vi "1-Tap 8-bit Camera with Bayer (FPGA).vi"() -> ()   [LabVIEW 2012]
doc: "This is the FPGA VI for the 1-Tap 8-Bit Camera with Bayer example. This example demonstrates how to acquire images from a 1-tap, 8-bit, base configuration, Camera Link camera, with a color sensor and transfer the decoded images to the host via a DMA FIFO.\n\nThis example also demonstrates the use of third-party IP imported into the LabVIEW project as a CLIP. In this case, the imported CLIP comes from an FPGA netlist and performs the Bayer color decoding to convert the incoming 8-bit Bayer images into 24-bit RGB images in real time.\n\nAdditionally, the example demonstrates the serial server, which allows third-party camera configuration utilities to communicate with the camera using the Camera Link serial interface while this VI is running."
uses:
  Common/CL Signal Mapping.ctl
  Common/CL Configuration.ctl
  <vilib>/Platform/TimedLoop/XDataNode/timing_clust.ctl
  <vilib>/Platform/TimedLoop/XDataNode/nitl_modes.ctl
  <vilib>/Platform/TimedLoop/XDataNode/wakeup.ctl
  <vilib>/rvi/eio/common/nirviEmuTemplateMethod_errors.vi
  <vilib>/rvi/Emulation/niFpgaSctlEmulationRegisterWithScheduler.vi
  <vilib>/rvi/Emulation/niFpgaSctlEmulationScheduler.vi
  Common/CL Data to Pixels/1 Tap 8-Bit.vi
  <vilib>/rvi/interface/RandomDataEmulation/nirviRandomDataFPGAFIFO.vi
  <vilib>/rvi/interface/RandomDataEmulation/niFpgaRandomDataHandleErrors.vi
  <vilib>/rvi/Emulation/niFpgaSctlEmulationGlobalWrite.vi
  <vilib>/Platform/TimedLoop/XDataNode/XDataNode.xnode
  <vilib>/eio/EIONode/EIONode.xnode
  <vilib>/rvi/DataTransferAndStorage/Container/XNode/niFpgaContainer.xnode
  <vilib>/rvi/interface/RandomDataEmulation/nirviRandomDataFpgaReadWriteTemplate.vi
  <vilib>/Platform/TimedLoop/XDataNode/XDNodeRunTimeDep.lvlib
panel:
  in  "CL Config.Configuration":T1
  in  "CL Config.Signal Mapping":T2
  in  "CL Config.Line Scan":bool
  in  "CL Config.DVAL Active High":bool=TRUE
  in  "CL Config.LVAL Active High":bool=TRUE
  in  "CL Config.FVAL Active High":bool=TRUE
  in  "CL Config.Spare Active High":bool=TRUE
  in  "Bayer Decoder.Image Width":u16
  in  "Bayer Decoder.First Column Is Red":bool
  in  "Bayer Decoder.First Row Is Blue":bool
  in  "Acq Control.Line Scan Height":u32
  in  "Acq Control.Frames To Acq":u32
  in  "Acq Control.Acquire":bool
  in  "Acq Control.Cancel Acq":bool
  in  "Acq Control.Ignore DVAL":bool
  in  "Acq Control.Initialize":bool
  out "Acq Status.Acq In Progress":bool
  out "Acq Status.Clocks Per Line":u32
  out "Acq Status.Frames Acq'd":u32
  out "Acq Status.Lines Per Frame":u32
  out "Acq Status.DMA Write Timeout":bool
  out "Acq Status.Initialized":bool
  in  "UART.Baud Rate":u8
  in  "UART.Transmit":bool
  in  "UART.Tx Data":u8[](array[numeric])=[0, 0, 0, 0, 0, 0, 0, 0, 0, 0] format="%02x"
  in  "UART.Set Baud Rate":bool
  in  "UART.Byte Mode":bool=TRUE
  out "UART.Rx Ready":bool
  out "UART.Break Indicator":bool
  out "UART.Framing Error":bool
  out "UART.Overrun Error":bool
  out "UART.Tx Ready":bool
  out "UART.Rx Data":u8 format="%02x"
  in  "UART.Receive":bool
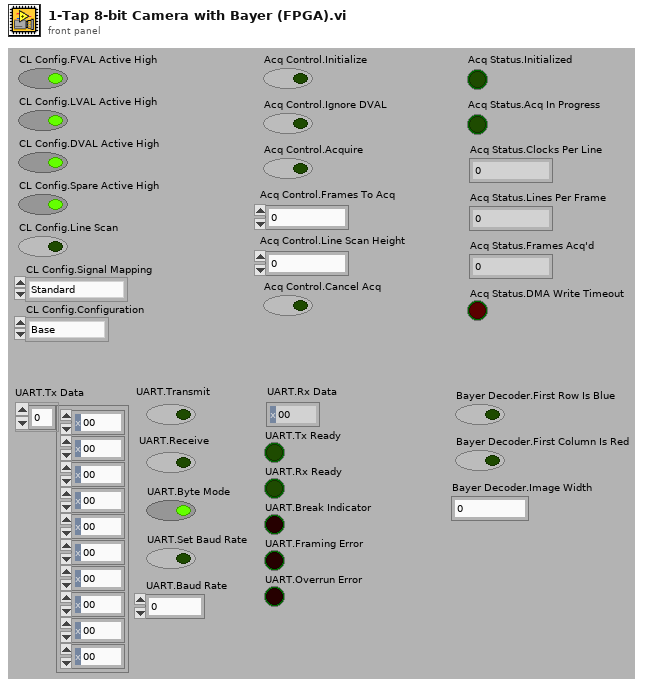
[diagram p1: front panel]
types:
  T1 = typedef "CL Configuration.ctl" = enum8{"Base", "Medium", "Full"}
  T2 = typedef "CL Signal Mapping.ctl" = enum8{"Standard", "Basler 10-tap", "Vosskühler 10-tap"}
  T3 = typedef "XDNodeRunTimeDep.lvlib/timing_clust.ctl" = cluster{"Expected End [f-1]":u64, "Actual End [f-1]":u64, "Finished Late? [f-1]":bool, "Expected End [i-1]":u64, "Actual End [i-1]":u64, "Finished Late? [i-1]":bool, "Expected Start [i]":u64, "Actual Start [i]":u64, "Expected Start [f]":u64, "Actual Start [f]":u64, "Source Name":string, "Structure Name":string, "Period":i64, "Deadline":i64, "Offset":i64, "Start":i64, "Priority":i32, "Timeout":i32, "Mode":T4, "Wakeup Reason":T5, "Error":errorcluster, "Source Type":string, "Secondary Source Type":string, "Global End Time":u64, "Global Start Time":u64, "Frame Duration":u64, "Iteration Duration":u64, "Assigned CPU":i32, "I/O Scan Engine Mode":u32}
  T4 = typedef "XDNodeRunTimeDep.lvlib/nitl_modes.ctl" = enum32{"No Change", "Process missed periods, maintain original phase", "Discard missed periods, maintain original phase", "Process missed periods, ignore original phase", "Discard missed periods, ignore original phase"}
  T5 = typedef "XDNodeRunTimeDep.lvlib/wakeup.ctl" = enum32{"Normal", "Aborted", "Asynchronous wakeup", "Timing source error", "Timed loop error", "Timeout"}
  T6 = cluster{"Enables Valid":bool, "Frame Valid":bool, "Line Valid":bool, "Data Valid":bool}
  T7 = cluster{"Tx Data":u8[], "Transmit":bool, "Receive":bool, "Byte Mode":bool, "Set Baud Rate":bool, "Baud Rate":u8}
  T8 = cluster{"Rx Data":u8, "Turn Off Transmit":bool, "Turn Off Receive":bool, "Turn Off Set Baud Rate":bool, "Tx Ready":bool, "Rx Ready":bool, "Break Indicator":bool, "Framing Error":bool, "Overrun Error":bool}
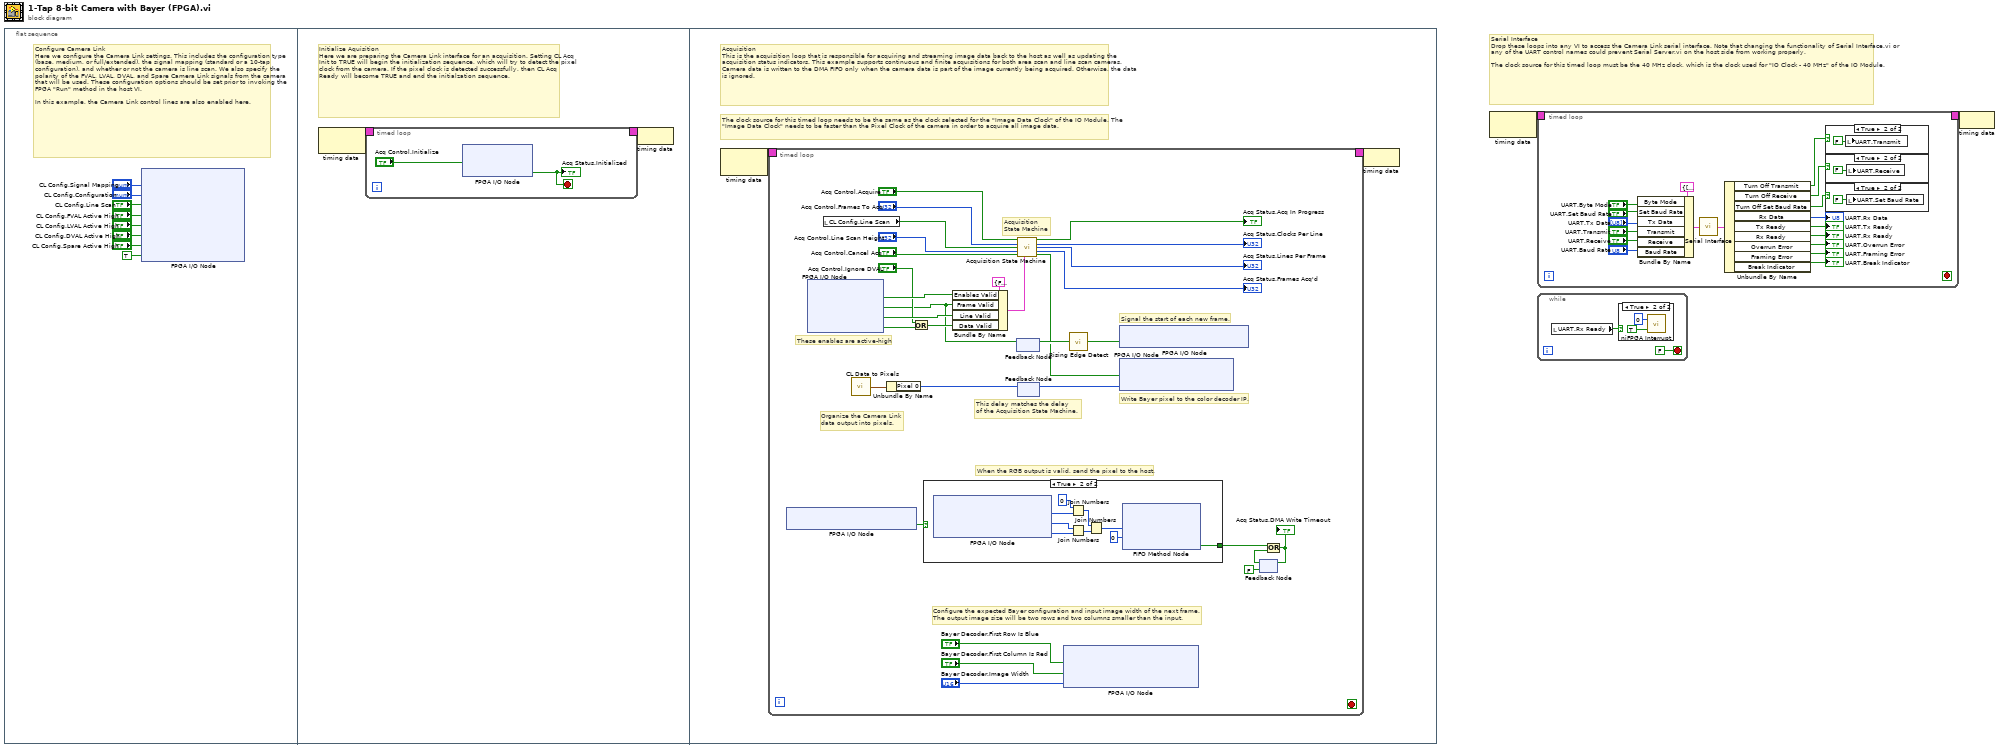
[diagram p0: block diagram]
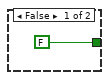
[diagram p6: hidden frame]
diagram:
  # "Serial Interface\nDrop these loops into any VI to access the Camera Link serial interface. Note that changing the functionality of Serial Interface.vi or any of the UART control names could prevent Serial Server.vi on the host side from working properly.\n\nThe clock source for this timed loop must be the 40 MHz clock, which is the clock used for \"IO Clock - 40 MHz\" of the IO Module."
  n1 = flat-sequence {
    frame #0 {
      # "Configure Camera Link\nHere we configure the Camera Link settings. This includes the configuration type (base, medium, or full/extended), the signal mapping (standard or a 10-tap configuration), and whether or not the camera is line scan. We also specify the polarity of the FVAL, LVAL, DVAL, and Spare Camera Link signals from the camera that will be used. These configuration options should be set prior to invoking the FPGA \"Run\" method in the host VI.\n\nIn this example, the Camera Link control lines are also enabled here."
      n2 = xnode "FPGA I/O Node"("CL Set Signal Mapping"="CL Config.Signal Mapping", "CL Set Configuration"="CL Config.Configuration", "CL Set Line Scan"="CL Config.Line Scan", "CL Set FVAL Active High"="CL Config.FVAL Active High", "CL Set LVAL Active High"="CL Config.LVAL Active High", "CL Set DVAL Active High"="CL Config.DVAL Active High", "CL Set Spare Active High"="CL Config.Spare Active High", "CL Control Enable"=TRUE ("IO Module\\CL Control Enable")) -> ()  [unwired: 8 in, 8 out]
    }
    frame #1 {
      # "Initialize Aquisition\nHere we are preparing the Camera Link interface for an acquisition. Setting CL Acq Init to TRUE will begin the initialization sequence, which will try to detect the pixel clock from the camera. If the pixel clock is detected successfully, then CL Acq Ready will become TRUE and end the initialzation sequence."
      n3 = node-c288() -> (w12:T3)  [unwired: 1 out]
      n4 = timed-loop {
        timing: w12 -> [_]
        timing-out: [_] -> w11
        stop <- w13 stop-if-true
        n5 = xnode "FPGA I/O Node"("CL Acq Init"="Acq Control.Initialize") -> ("CL Acq Ready"=w13:bool)  [unwired: 2 in, 2 out]
        "Acq Status.Initialized" <- w13
      }
      n6 = node-c288(w11) -> ()
    }
    frame #2 {
      # "The clock source for this timed loop needs to be the same as the clock selected for the \"Image Data Clock\" of the IO Module. The \"Image Data Clock\" needs to be faster than the Pixel Clock of the camera in order to acquire all image data."
      # "Acquisition\nThis is the acquisition loop that is responsible for acquiring and streaming image data back to the host as well as updating the acquisition status indicators. This example supports continuous and finite acquisitions for both area scan and line scan cameras. Camera data is written to the DMA FIFO only when the camera data is part of the image currently being acquired. Otherwise, the data is ignored."
      n7 = node-c288() -> (w20:T3)  [unwired: 1 in]
      n8 = timed-loop {
        timing: w20 -> [_]
        timing-out: [_] -> w19
        stop <- _ stop-if-true
        # "Configure the expected Bayer configuration and input image width of the next frame.\nThe output image size will be two rows and two columns smaller than the input."
        # "When the RGB output is valid, send the pixel to the host."
        # "Write Bayer pixel to the color decoder IP."
        # "Signal the start of each new frame."
        # "Organize the Camera Link\ndata output into pixels."
        # "These enables are active-high"
        # "This delay matches the delay\nof the Acquisition State Machine."
        # "Acquisition\nState Machine"
        n9 = xnode "FPGA I/O Node"() -> ("Bayer Decoder\\RGB Output Valid"=w30:bool)  [unwired: 1 in, 1 out]
        n10 = xnode "FPGA I/O Node"() -> ("CL Output Valid"=w39:bool, "CL Frame Valid"=w27:bool, "CL Line Valid"=w38:bool, "CL Data Valid"=w35:bool)  [unwired: 4 in, 4 out]
        n11 = local read "CL Config.Line Scan"() -> (w32:bool)
        n12 = call-poly "CL Data to Pixels.vi"() -> ("Pixels"=w51:cluster{"Pixel 0":u8})  [unwired: 1 in]
        n13 = Unbundle By Name(w51) -> ("Pixel 0"=w50:u8)
        n14 = Or(x="Acq Control.Ignore DVAL", y=w35) -> (x .or. y?=w34:bool)
        n15 = case shown="True" w30 {
          tunnel: [FALSE ("Timed Out?") w54] -> w29
          frame False {
          }
          frame True {
            n16 = xnode "FPGA I/O Node"() -> ("Bayer Decoder\\Blue Output"=w58:u8, "Bayer Decoder\\Green Output"=w57:u8, "Bayer Decoder\\Red Output"=w61:u8)  [unwired: 3 in, 3 out]
            n17 = Join Numbers(hi=u8 0, lo=w58) -> ((hi.lo)=w59:u16)
            n18 = Join Numbers(hi=w57, lo=w61) -> ((hi.lo)=w60:u16)
            n19 = Join Numbers(hi=w59, lo=w60) -> ((hi.lo)=w55:u32)
            n20 = xnode ("FIFO Method Node")("Element"=w55, "Timeout"=0) -> ("Timed Out?"=w54:bool)  [unwired: 1 in, 1 out]
          }
        }
        n21 = Bundle By Name(cluster=T6 {"Enables Valid"=FALSE, "Frame Valid"=FALSE, "Line Valid"=FALSE, "Data Valid"=FALSE} ("Enables"), "Enables Valid"=w39, "Frame Valid"=w27, "Line Valid"=w38, "Data Valid"=w34) -> (w37:T6)
        n22 = feedback #1() -> (w26:bool)  [unwired: 1 in]
        n23 = feedback-in #1(w27) -> ()
        n24 = feedback-in #2(w50) -> ()
        n25 = feedback #2() -> (w28:u8)  [unwired: 1 in]
        n26 = call "Acquisition State Machine.vi"("Acquire"="Acq Control.Acquire", "Frames to Acquire"="Acq Control.Frames To Acq", "Line Scan"=w32, "Line Scan Height"="Acq Control.Line Scan Height", "Cancel Acq"="Acq Control.Cancel Acq", "Enables"=w37) -> ("Acq In Progress"=→"Acq Status.Acq In Progress":bool, "Num Clocks Per Line"=→"Acq Status.Clocks Per Line":u32, "Num Lines Per Frame"=→"Acq Status.Lines Per Frame":u32, "Num Frames Acq'd"=→"Acq Status.Frames Acq'd":u32, "Capture Cycle"=w25:bool)  [unwired: 4 in, 1 out]
        n27 = xnode "FPGA I/O Node"("Bayer Decoder\\First Row Is Blue"="Bayer Decoder.First Row Is Blue", "Bayer Decoder\\First Column Is Red"="Bayer Decoder.First Column Is Red", "Bayer Decoder\\Image Width"="Bayer Decoder.Image Width") -> ()  [unwired: 3 in, 3 out]
        n28 = call "Rising Edge Detect.vi"("Input"=w26) -> ("Pulse"=w24:bool)  [unwired: 4 in]
        n29 = xnode "FPGA I/O Node"("Bayer Decoder\\New Frame Pulse"=w24) -> ()  [unwired: 1 in, 1 out]
        n30 = xnode "FPGA I/O Node"("Bayer Decoder\\Write Enable"=w25, "Bayer Decoder\\Pixel In"=w28) -> ()  [unwired: 2 in, 2 out]
        n31 = feedback #3(FALSE) -> (w48:bool)
        n32 = Or(x=w29, y=w48) -> (x .or. y?=w47:bool)
        "Acq Status.DMA Write Timeout" <- w47
        n33 = feedback-in #3(w47) -> ()
      }
      n34 = node-c288(w19) -> ()
    }
  }
  n35 = node-c288() -> (w2:T3)  [unwired: 1 out]
  n36 = timed-loop {
    timing: w2 -> [_]
    timing-out: [_] -> w1
    stop <- _ stop-if-true
    n37 = Bundle By Name(cluster=T7 {"Tx Data"=[0, 0, 0, 0, 0, 0, 0, 0, 0, 0], "Transmit"=FALSE, "Receive"=FALSE, "Byte Mode"=TRUE, "Set Baud Rate"=FALSE, "Baud Rate"=0} ("UART Inputs"), "Byte Mode"="UART.Byte Mode", "Set Baud Rate"="UART.Set Baud Rate", "Tx Data"="UART.Tx Data", "Transmit"="UART.Transmit", "Receive"="UART.Receive", "Baud Rate"="UART.Baud Rate") -> (w66:T7)
    n38 = call "Serial Interface.vi"("UART Inputs"=w66) -> ("UART Outputs"=w78:T8)
    n39 = Unbundle By Name(w78) -> ("Turn Off Transmit"=w71:bool, "Turn Off Receive"=w72:bool, "Turn Off Set Baud Rate"=w68:bool, "Rx Data"=→"UART.Rx Data":u8, "Tx Ready"=→"UART.Tx Ready":bool, "Rx Ready"=→"UART.Rx Ready":bool, "Overrun Error"=→"UART.Overrun Error":bool, "Framing Error"=→"UART.Framing Error":bool, "Break Indicator"=→"UART.Break Indicator":bool)
    n40 = case shown="True" w71 {
      frame False {
      }
      frame True {
        n41 = local write "UART.Transmit"(FALSE ("UART.Transmit")) -> ()
      }
    }
    n42 = case shown="True" w72 {
      frame False {
      }
      frame True {
        n43 = local write "UART.Receive"(FALSE ("UART.Receive")) -> ()
      }
    }
    n44 = case shown="True" w68 {
      frame False {
      }
      frame True {
        n45 = local write "UART.Set Baud Rate"(FALSE ("UART.Receive")) -> ()
      }
    }
  }
  n46 = while {
    stop <- FALSE stop-if-true
    n47 = local read "UART.Rx Ready"() -> (w90:bool)
    n48 = case shown="True" w90 {
      frame False {
      }
      frame True {
        n49 = call <vilib>:"niFPGA Interrupt.vi"("Wait Until Cleared (F)"=TRUE ("Wait Until Cleared"), "IRQ Number (0)"=u8 0 ("IRQ Number")) -> ()  [unwired: 1 in]
      }
    }
  }
  n50 = node-c288(w1) -> ()
